vi "Ophir range.vi"() -> ()   [LabVIEW 2012]
doc: "Terminal.vi\nUse the terminal to send commands to instrument.\nThe terminal displays the answer in Nova2 Response\nVersion 1.00\nLast Updated 16 March 2005\n\nYou must select Communication Protocol : USB or RS232\nwhen USB is default.\n\nCommand : String\nInsert here the Command you want to send to Nova2 \n\nDevice Response : String\nDisplay the device's response to the sended Command \n\nSend Command : Boolean button\nPush it to send the command written in Command.\nOr press Enter\n\nStop Terminal : Boolean button\nPush it to stop the Terminal Loop\nOr press Escape"
panel:
  out "Command 2":string
  out "String":string="Be sure to run the SwapINF utility to enable communication with the USBI, Vega and Nova2 devices in USB"
  in  "GPIB Address (10)":string="10"
  in  "Select Communication Protocol":u16(ring)=2 items=["USB - Nova2", "USB - Vega", "USB - USBI", "RS232", "GPIB"]
  in  "usb channel":i16
  out "VISA resource name":refnum<visa-resource-name>="USB0::0x0BD3::0x0333::NI-VISA-0::RAW"
  in  "Baud Rate (3:9600)":i16(ring)=4 items=["300", "1200", "4800", "9600", "19200", "38400"]
  in  "Port Number (default 2)":i16=1 min=0 max=20
  out "error out":errorcluster
  in  "Command":string
  out "Device Response":string="\r\n"
  in  "error in (no error)":errorcluster
  # "Terminal"
  # "GPIB -"
  # "USB -"
  # "RS232  -"
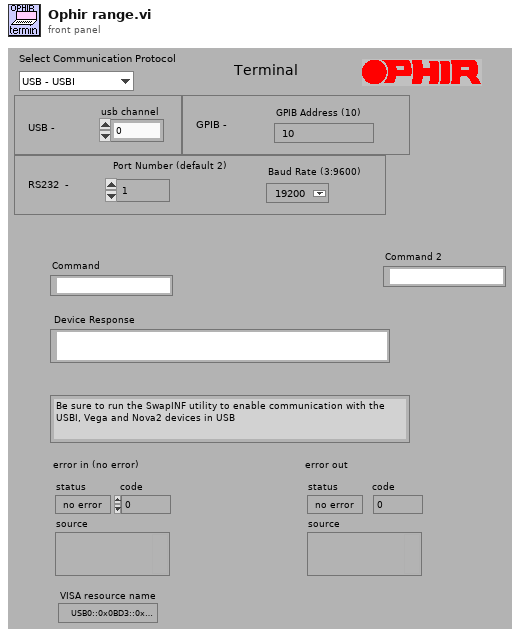
[diagram p1: front panel]
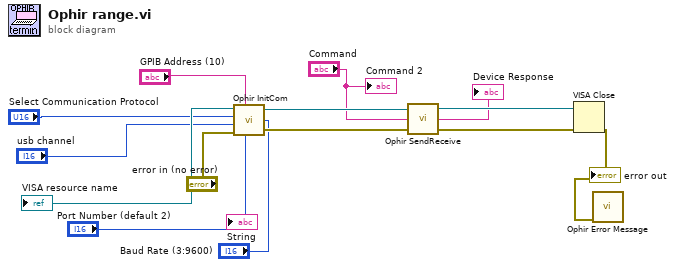
[diagram p0: block diagram]
diagram:
  n1 = call "Ophir InitCom.vi"("GPIB Address (10)"="GPIB Address (10)", "communication"="Select Communication Protocol", "Numeric"="usb channel", "Port Number (default 2)"="Port Number (default 2)", "error in (no error)"="error in (no error)", "Baud Rate (3:9600)"="Baud Rate (3:9600)") -> ("Visa Session"=→"VISA resource name":refnum<visa-resource-name>, "dup Visa Session"=w11:refnum<visa-resource-name>, "error out"=w10:errorcluster)
  n2 = call "Ophir SendReceive.vi"("error in (no error)"=w10, "Command"="Command", "Visa Session"=w11) -> ("error out"=w14:errorcluster, "Frame Output"=→"Device Response":string, "dup Visa Session"=w13:refnum<visa-resource-name>)
  n3 = VISA Close(VISA resource name=w13, error in (no error)=w14) -> (error out=w9:errorcluster)
  "error out" <- w9
  n4 = call "Ophir Error Message.vi"("error in (no error)"=w9) -> ()  [unwired: 3 in, 4 out]
  "Command 2" <- "Command"
